vi "OpenClipboard.vi"(4 "error in (no error)":errorcluster) -> (0 "error out":errorcluster)   [LabVIEW 2011]
uses:
  user32.dll
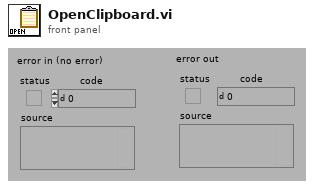
[diagram p1: front panel]
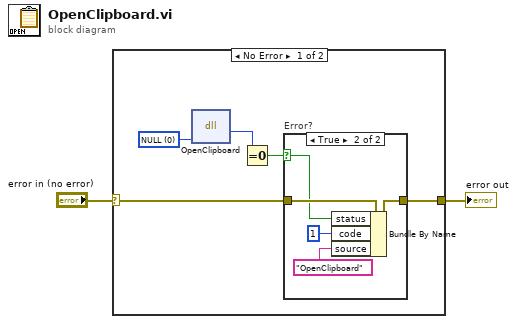
[diagram p0: block diagram]
diagram:
  n1 = case shown="No Error" "error in (no error)" {
    selector: "error in (no error)" -> [w3 w14]
    tunnel: [w7 w14] -> w2
    frame No Error {
      w4 = u32 0 items=["NULL"]
      n2 = dll-call lib="User32.dll" fn="OpenClipboard" label="unsigned long OpenClipboard(\n    unsigned long hWndNewOwner);"("hWndNewOwner"=w4) -> (w5:u32)  [unwired: 4 in, 2 out]
      n3 = Equal To 0?(x=w5) -> (x = 0?=w6:bool)
      n4 = case "Error?" shown="True" w6 {
        selector: w6 -> [_ w12]
        tunnel: w3 -> [w8 w13]
        tunnel: [w8 w9] -> w7
        frame False {
        }
        frame True {
          n5 = Bundle By Name(cluster=w13, "status"=w12, "code"=1, "source"="OpenClipboard") -> (w9:errorcluster)
        }
      }
    }
    frame Error {
    }
  }
  "error out" <- w2
